vi "Angular Velocity Controler.vi"(7 "reinitialize? (F)":bool, 8 "Command Heading":dbl, 10 "PID gains":cluster{"P":dbl, "I":dbl, "D":dbl}, 11 "Period":i64) -> (3 "VAng_Cmd":dbl(slide) scale=-10.0..10.0)   [LabVIEW 2012]
uses:
  <vilib>/addons/control/pid/pid.llb/PID Structure Conversion (DBL).vi
  <vilib>/addons/control/pid/pid.llb/PID Advanced (DBL).vi
  <vilib>/addons/control/pid/NI_PID_pid.lvlib
panel:
  in  "x":dbl
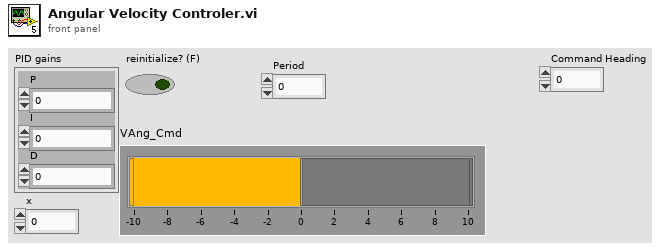
[diagram p1: front panel]
types:
  T1 = enum16{"Academic (Standard)", "Parallel", "Series"}
  T2 = cluster{"proportional gain (Kc)":dbl, "integral time (Ti, min)":dbl, "derivative time (Td, min)":dbl}
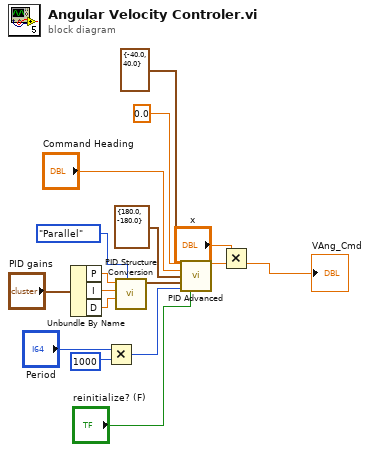
[diagram p0: block diagram]
diagram:
  n1 = Unbundle By Name("PID gains") -> ("P"=w11:dbl, "I"=w12:dbl, "D"=w13:dbl)
  n2 = Multiply(x="Period", y=i64 1000) -> (x*y=w7:i64)
  n3 = call-poly <vilib>:"PID Structure Conversion.vi"("PID structure"=T1."Parallel", "derivative"=w13, "integral"=w12, "proportional"=w11) -> ("PID gains"=w10:T2)  [unwired: 7 in]
  n4 = call-poly <vilib>:"PID Advanced.vi"("setpoint"=0.0, "output range"=cluster{"output high":dbl, "output low":dbl} {"output high"=-40.0, "output low"=40.0}, "process variable"="Command Heading", "setpoint range"=cluster{"setpoint high":dbl, "setpoint low":dbl} {"setpoint high"=180.0, "setpoint low"=-180.0}, "PID gains"=w10, "dt (s)"=w7, "reinitialize? (F)"="reinitialize? (F)") -> ("output"=w4:dbl)  [unwired: 7 in, 1 out]
  n5 = Multiply(x="x", y=w4) -> (x*y=→"VAng_Cmd":dbl)
